vi "Initialize.vi"(8 "error in":errorcluster, 9 "Number of Channels":u32=1, 10 "Plugin Name":string, 11 "Resistance Control in":refnum<class "Resistance Control.lvclass">) -> (0 "error out":errorcluster, 3 "Resistance Control out":refnum<class "Resistance Control.lvclass">)   [LabVIEW 2023, in "Resistance Control.lvclass"]
uses:
  Resistance Control.lvclass
  Resistance Control.lvclass/Resistance Control.ctl
  <vilib>/ADAS Replay HIL/Channels/Tag Wrapper/Polymorphic/Open Consumer Tag (Double).vi
  <vilib>/ADAS Replay HIL/Channels/Tag Wrapper/Polymorphic/Open Producer Tag (Double).vi
  <vilib>/ADAS Replay HIL/Channels/Tag Wrapper/Polymorphic/Open Consumer Tag (Double).vi/bacb721e-673a-491a-accd-959f2e1f334e.vi
  <vilib>/ADAS Replay HIL/Channels/Tag Wrapper/Polymorphic/Open Producer Tag (Double).vi/45cd6eaa-a1ce-41a4-8aba-62a49d103d7e.vi
  <vilib>/ADAS Replay HIL/Channels/Tag Wrapper/Polymorphic/Open Consumer Tag (Double).vi/bacb721e-673a-491a-accd-959f2e1f334e.vi/c28b0ead-42ad-4072-80a2-aca7f2bd7ce3.vi
  <vilib>/ADAS Replay HIL/Channels/Tag Wrapper/Polymorphic/Open Producer Tag (Double).vi/45cd6eaa-a1ce-41a4-8aba-62a49d103d7e.vi/c28b0ead-42ad-4072-80a2-aca7f2bd7ce3.vi
  <vilib>/ADAS Replay HIL/AdasHilServices/AdasHilServices Fill In Error Info Ex.vi
  <vilib>/ADAS Replay HIL/Channels/Tag Wrapper/Tag Wrapper.lvlib
  Utilities/Utilities.lvlib
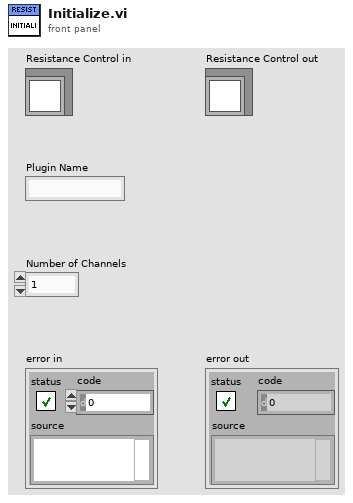
[diagram p1: front panel]
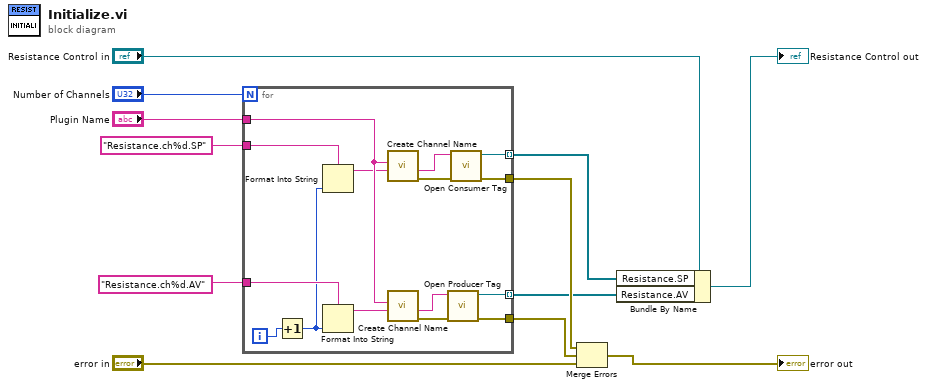
[diagram p0: block diagram]
diagram:
  n1 = for {
    N: "Number of Channels" -> [_]
    tunnel: "Resistance.ch%d.SP" ("Consumer Tag") -> [w18]
    tunnel: "Plugin Name" -> [w26]
    tunnel: "Resistance.ch%d.AV" ("Producer Tag") -> [w17]
    tunnel: [w22] -> w7
    tunnel: [w21] -> w6
    tunnel: [w14] -> w2 mode=indexing
    tunnel: [w13] -> w1 mode=indexing
    i -> [w16]
    n2 = Increment(x=w16) -> (x+1=w15:i32)
    n3 = Format Into String(format string=w18, w15) -> (resulting string=w20:string)  [unwired: 2 in, 1 out]
    n4 = Format Into String(format string=w17, w15) -> (resulting string=w19:string)  [unwired: 2 in, 1 out]
    n5 = call "Create Channel Name.vi"("Channel Name"=w20, "Plugin Name"=w26) -> ("error out"=w24:errorcluster, "Data Channel Name"=w27:string)  [unwired: 8 in]
    n6 = call "Create Channel Name.vi"("Channel Name"=w19, "Plugin Name"=w26) -> ("error out"=w23:errorcluster, "Data Channel Name"=w25:string)  [unwired: 8 in]
    n7 = call-poly <vilib>:"Open Producer Tag.vi"("error in"=w23, "Channel Name"=w25) -> ("error out"=w21:errorcluster, "ADAS HIL Channel"=w13:refnum<k21>)  [unwired: 8 in]
    n8 = call-poly <vilib>:"Open Consumer Tag.vi"("error in"=w24, "Channel Name"=w27) -> ("error out"=w22:errorcluster, "ADAS HIL Channel"=w14:refnum<k21>)  [unwired: 8 in]
  }
  n9 = Merge Errors(w7, w6, "error in") -> (→"error out":errorcluster)
  n10 = Bundle By Name(cluster="Resistance Control in", "Resistance.SP"=w2, "Resistance.AV"=w1) -> (→"Resistance Control out":refnum<class "Resistance Control.lvclass">)
